vi "Calculate_Dewpoint.vi"(1 "Outside humidity":sgl, 2 "Outside temperature (F)":sgl format="%#.1f") -> (0 "Dewpoint (C)":sgl format="%#.1f")   [LabVIEW 2012]
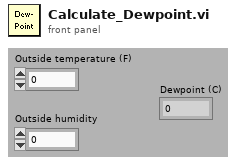
[diagram p1: front panel]
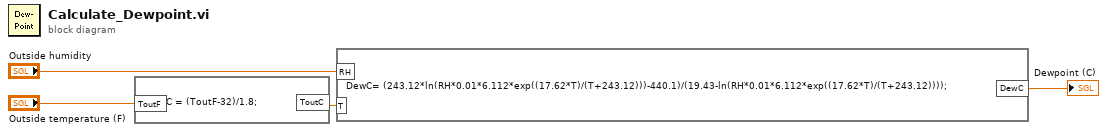
[diagram p0: block diagram]
diagram:
  n1 = formula code="ToutC = (ToutF-32)/1.8;"("ToutF"="Outside temperature (F)") -> ("ToutC"=w2:dbl)
  n2 = formula code="DewC= (243.12*ln(RH*0.01*6.112*exp((17.62*T)/(T+243.12)))-440.1)/(19.43-ln(RH*0.01*6.112*exp((17.62*T)/(T+243.12))));"("RH"="Outside humidity", "T"=w2) -> ("DewC"=→"Dewpoint (C)":dbl)
